vi "Set Filepath.vi"(8 "error in":errorcluster, 10 "Filepath":path, 11 "FileHandler in":refnum<class "FileHandler.lvclass">) -> (0 "error out":errorcluster, 3 "FileHandler out":refnum<class "FileHandler.lvclass">)   [LabVIEW 2016, in "hse-logger.lvlib" / "FileHandler.lvclass"]
uses:
  FileHandler.lvclass
  FileHandler.lvclass/FileHandler.ctl
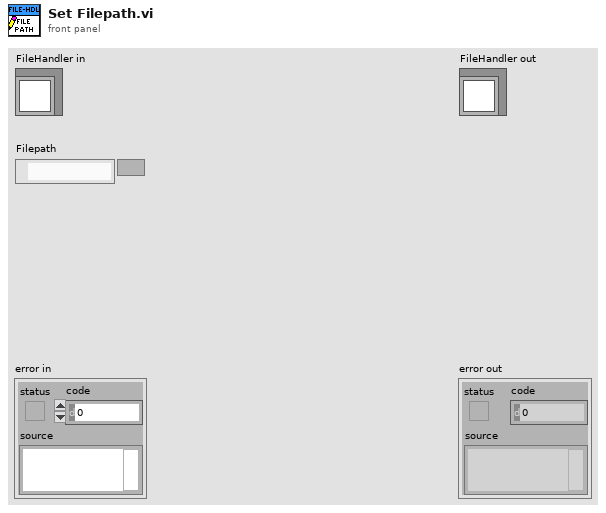
[diagram p1: front panel]
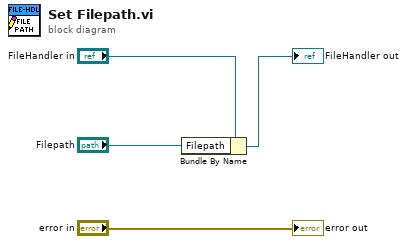
[diagram p0: block diagram]
diagram:
  n1 = Bundle By Name(cluster="FileHandler in", "Filepath"="Filepath") -> (→"FileHandler out":refnum<class "FileHandler.lvclass">)
  "error out" <- "error in"
